vi "Com Port Connection.vi"(8 "error in":errorcluster, 11 "Com Port In":refnum<visa-resource-name>) -> (0 "error out":errorcluster, 3 "Com Port Out":refnum<visa-resource-name>)   [LabVIEW 2018]
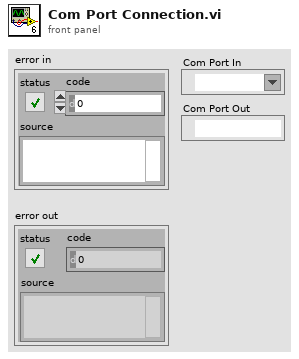
[diagram p1: front panel]
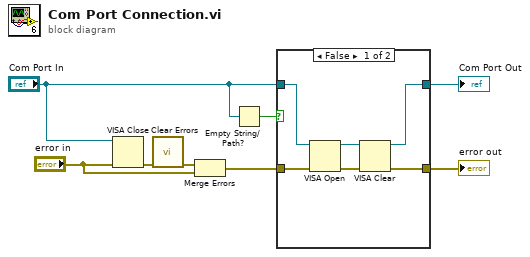
[diagram p0: block diagram]
diagram:
  n1 = VISA Close(VISA resource name="Com Port In", error in (no error)="error in") -> (error out=w8:errorcluster)
  n2 = call <vilib>:"Clear Errors.vi"("error in (no error)"=w8) -> ("error out"=w6:errorcluster)  [unwired: 5 in, 1 out]
  n3 = Merge Errors(w6, "error in") -> (w4:errorcluster)
  n4 = Empty String/Path?(string/path="Com Port In") -> (empty?=w3:bool)
  n5 = case shown="False" w3 {
    tunnel: [w12 w15] -> w7
    tunnel: w4 -> [w11 w15]
    tunnel: "Com Port In" -> [w10 w16]
    tunnel: [w9 w16] -> w2
    frame False {
      n6 = VISA Open(error in (no error)=w11, VISA resource name=w10) -> (VISA resource name=w13:refnum<visa-resource-name>, error out=w14:errorcluster)  [unwired: 3 in]
      n7 = VISA Clear(VISA resource name=w13, error in (no error)=w14) -> (VISA resource name out=w9:refnum<visa-resource-name>, error out=w12:errorcluster)
    }
    frame True {
    }
  }
  "error out" <- w7
  "Com Port Out" <- w2
